vi "start.vi"() -> ()   [LabVIEW 2014]
uses:
  <vilib>/Utility/error.llb/DialogType.ctl
panel:
  in  "退出":bool
  in  "other":bool
  in  "CAN":bool
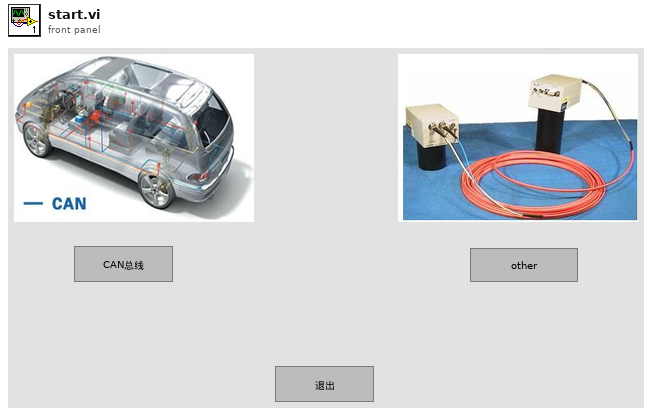
[diagram p1: front panel]
types:
  T1 = enum32{"Invalid", "Standard", "Closed", "Hidden", "Minimized", "Maximized"}
  T2 = typedef "DialogType.ctl" = u16
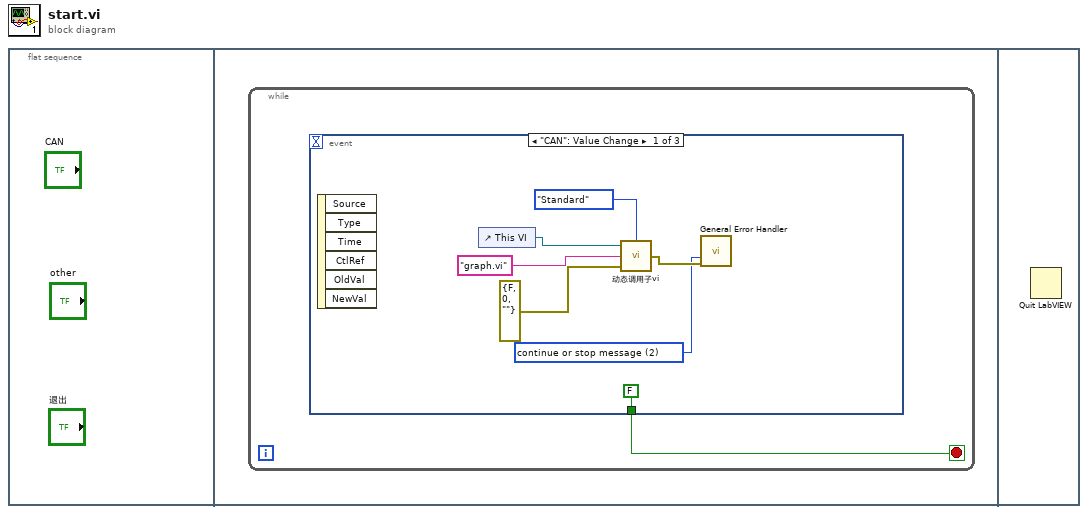
[diagram p0: block diagram]
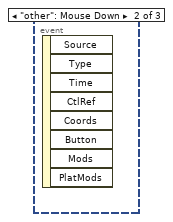
[diagram p2: hidden frame]
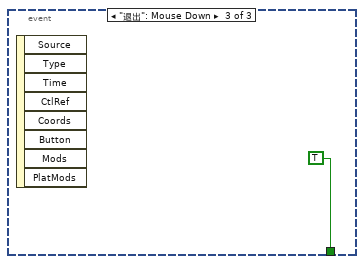
[diagram p3: hidden frame]
diagram:
  n1 = flat-sequence {
    frame #0 {
    }
    frame #1 {
      n2 = while {
        stop <- w1 stop-if-true
        n3 = event shown="[0] \"CAN\": Value Change" {
          selector: _ -> [_ _ _]
          dyn-events: _ -> [_ _ _]
          timeout: _ -> [_ _ _]
          tunnel: [FALSE _ TRUE] -> w1
          event "CAN": Value Change {
            w4 = T2 2 items=["no dialog", "OK message", "continue or stop message", "OK message + warnings", "continue/stop + warnings"] ("type of dialog (OK msg:1)")
            n4 = event-data() -> ()  [unwired: 1 in, 6 out]
            n5 = control-ref of="This VI"() -> (w8:refnum<vi>)
            n6 = call "动态调用子vi.vi"("Front Panel Window:State"=T1."Standard", "error in (no error)"=errorcluster {"status"=FALSE, "code"=0, "source"=""}, "被调用的子vi"="graph.vi", "VI Refnum"=w8) -> ("error out"=w5:errorcluster)
            n7 = call <vilib>:"General Error Handler.vi"("type of dialog (OK msg:1)"=w4, "error in (no error)"=w5) -> ()  [unwired: 9 in, 5 out]
          }
          event "other": Mouse Down {
            n8 = event-data() -> ()  [unwired: 1 in, 8 out]
          }
          event "退出": Mouse Down {
            n9 = event-data() -> ()  [unwired: 1 in, 8 out]
          }
        }
      }
    }
    frame #2 {
      n10 = Quit LabVIEW() -> ()  [unwired: 1 in]
    }
  }
